vi "Timing_just64bitnumbercounting.vi"(11 "initial value":u64) -> (3 "x+1":u64)   [LabVIEW 2012]
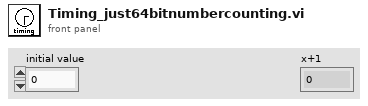
[diagram p1: front panel]
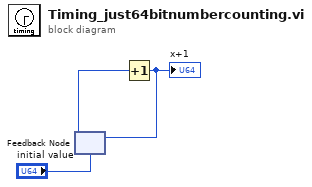
[diagram p0: block diagram]
diagram:
  n1 = feedback #1("initial value") -> (w3:u64)
  n2 = Increment(x=w3) -> (x+1=w1:u64)
  "x+1" <- w1
  n3 = feedback-in #1(w1) -> ()
